vi "Output Protection Status.vi"(8 "error in (no error)":errorcluster, 11 "VISA resource name":refnum<visa-resource-name>) -> (0 "error out":errorcluster, 1 "OCP Tripped":bool, 2 "OVP Tripped":bool, 3 "VISA resource name out":refnum<visa-resource-name>, 5 "OPP Tripped":bool)   [LabVIEW 2018, in "XP Power PLS600.lvlib"]
doc: "Reads the voltage, current, and power protection status. NOTE: Over-Voltage, Over-Current, and Over-Power are reported as errors by the Error Query. This VI will automatically call the Error Query and will decode the error to determine if any of the protection limits have been exceeded. You must manually clear the error if you wish to programmatically recover during runtime."
uses:
  XP Power PLS600.lvlib
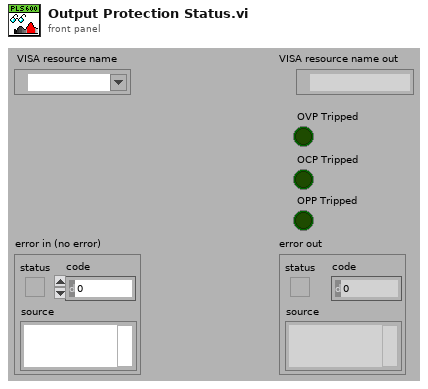
[diagram p1: front panel]
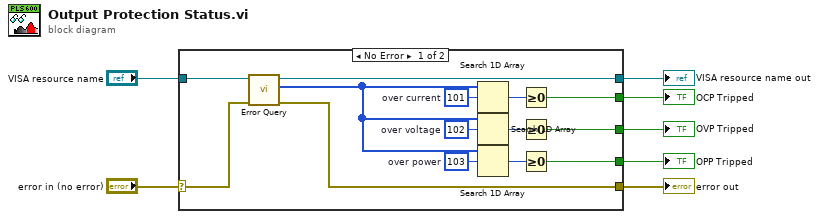
[diagram p0: block diagram]
diagram:
  n1 = case shown="No Error" "error in (no error)" {
    selector: "error in (no error)" -> [w9 w22]
    tunnel: [w21 w23] -> w7
    tunnel: "VISA resource name" -> [w20 w23]
    tunnel: [w8 w22] -> w5
    tunnel: [w13 _] -> w4
    tunnel: [w12 _] -> w3
    tunnel: [w11 _] -> w2
    frame No Error {
      w17 = 103  # over power
      w18 = 102  # over voltage
      w19 = 101  # over current
      n2 = call "Error Query.vi"("error in (no error)"=w9, "VISA resource name"=w20) -> ("error out"=w8:errorcluster, "Error Code"=w10:i32[], "VISA resource name out"=w21:refnum<visa-resource-name>)  [unwired: 6 in, 1 out]
      n3 = Search 1D Array(1D array=w10, element=w19) -> (index of element=w16:i32)  [unwired: 1 in]
      n4 = Search 1D Array(1D array=w10, element=w18) -> (index of element=w15:i32)  [unwired: 1 in]
      n5 = Search 1D Array(1D array=w10, element=w17) -> (index of element=w14:i32)  [unwired: 1 in]
      n6 = Greater Or Equal To 0?(x=w16) -> (x >= 0?=w13:bool)
      n7 = Greater Or Equal To 0?(x=w15) -> (x >= 0?=w12:bool)
      n8 = Greater Or Equal To 0?(x=w14) -> (x >= 0?=w11:bool)
    }
    frame Error {
    }
  }
  "VISA resource name out" <- w7
  "error out" <- w5
  "OVP Tripped" <- w3
  "OCP Tripped" <- w4
  "OPP Tripped" <- w2
